vi "IsStarboard.vi"(8 "error in (no error)":errorcluster, 10 "Boat Heading (Deg.)":dbl, 11 "Angle in":refnum<class "Angle.lvclass">) -> (0 "error out":errorcluster, 2 "IsStarboard":bool)   [LabVIEW 2012]
doc: "Take in angle, robot heading, returns a boolean \"Is Starboard\", 0 or 1"
uses:
  Angle.lvclass
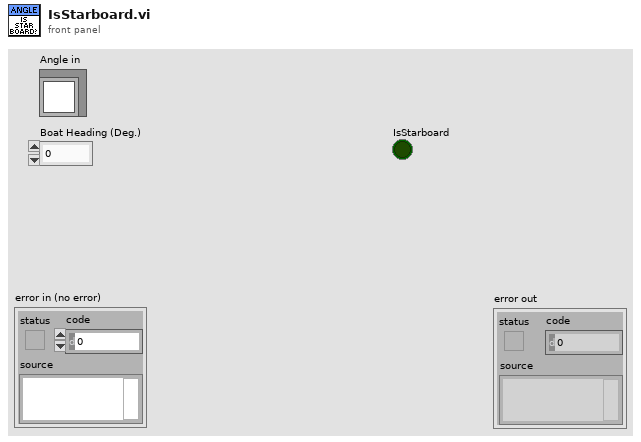
[diagram p1: front panel]
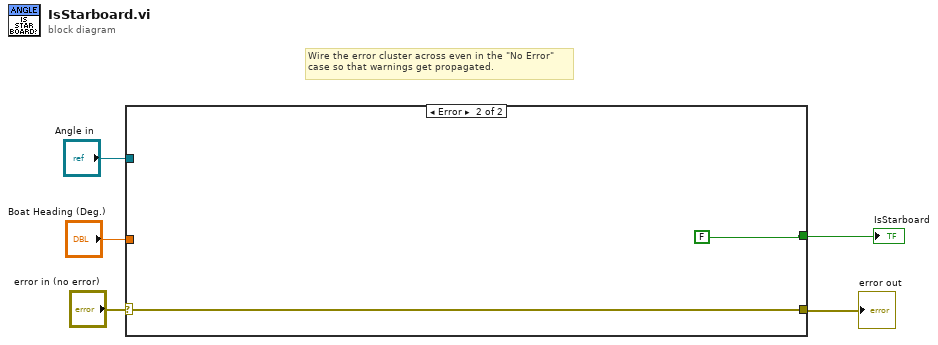
[diagram p0: block diagram]
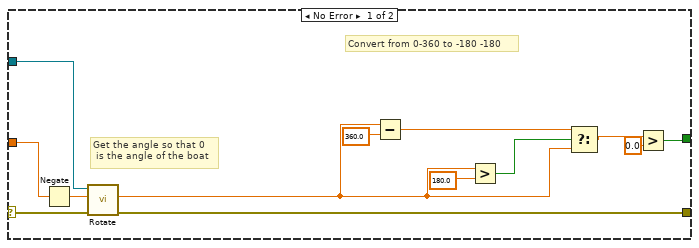
[diagram p2: hidden frame]
diagram:
  # "Wire the error cluster across even in the \"No Error\"\ncase so that warnings get propagated."
  n1 = case shown="Error" "error in (no error)" {
    selector: "error in (no error)" -> [w18 w20]
    tunnel: [w17 w20] -> w4
    tunnel: "Angle in" -> [w16 _]
    tunnel: [w7 FALSE] -> w2
    tunnel: "Boat Heading (Deg.)" -> [w9 _]
    frame No Error {
      # "Convert from 0-360 to -180 -180"
      # "Get the angle so that 0\n is the angle of the boat"
      n2 = Negate(x=w9) -> (-x=w10:dbl)
      n3 = call "Rotate.vi"("error in (no error)"=w18, "Rotation Angle (Deg.)"=w10, "Angle in"=w16) -> ("error out"=w17:errorcluster, "New Angle"=w11:dbl)  [unwired: 6 in, 1 out]
      n4 = Subtract(x=w11, y=360.0) -> (x-y=w13:dbl)
      n5 = Greater?(x=w11, y=180.0) -> (0:w15:bool)
      n6 = Select(t=w13, s=w15, f=w11) -> (s? t:f=w6:dbl)
      n7 = Greater?(x=w6, y=0.0) -> (0:w7:bool)
    }
    frame Error {
    }
  }
  "error out" <- w4
  "IsStarboard" <- w2
